vi "Data Display Manager.vi"(6 "Volt Channel":T1={"Index"=[], "Chl Name"=[], "Scale"=[], "Offset"=[], "Sample Rate"=100, "Device Name"="", "Channel"=""}, 7 "Enum":T2=enum."Config Data", 8 "error in":errorcluster, 9 "Raw Data":waveform(dbl)[](array[waveform]), 11 "Data Display Choice":T3) -> (0 "error out":errorcluster, 1 "Overall Mean":dbl[](array[numeric]), 2 "Mean per Second":dbl[](array[numeric]), 3 "VI Ref":refnum<vi>, 4 "Conditioned Data Out":waveform(dbl)[](array[waveform]))   [LabVIEW 2021]
doc: "This Vi has three functions:\nConfig Data - Reset Total Samples, Mean per Second and Overall Mean\nVolt Data - Display Data and calculate Mean per Second and Overall Mean\nDisplay Choice - Choose an appropriate displaying method and pass the chart or graph vi reference out."
uses:
  Control/Data Display Choice Enum.ctl
  Control/Data Display Manager Enum.ctl
  Control/Volt Chl.ctl
  Graph Abstract Class/Pass Ref and Receive Data -- Enum.ctl
  Graph Abstract Class/Graph Data -- cluster.ctl
  Graph Abstract Class/Display Abstract.lvclass
  Chart Class/Chart.lvclass
  Graph Class/Graph.lvclass
  <vilib>/Analysis/baseanly.llb/Mean (DBL).vi
  <vilib>/Analysis/NI_AALBase.lvlib
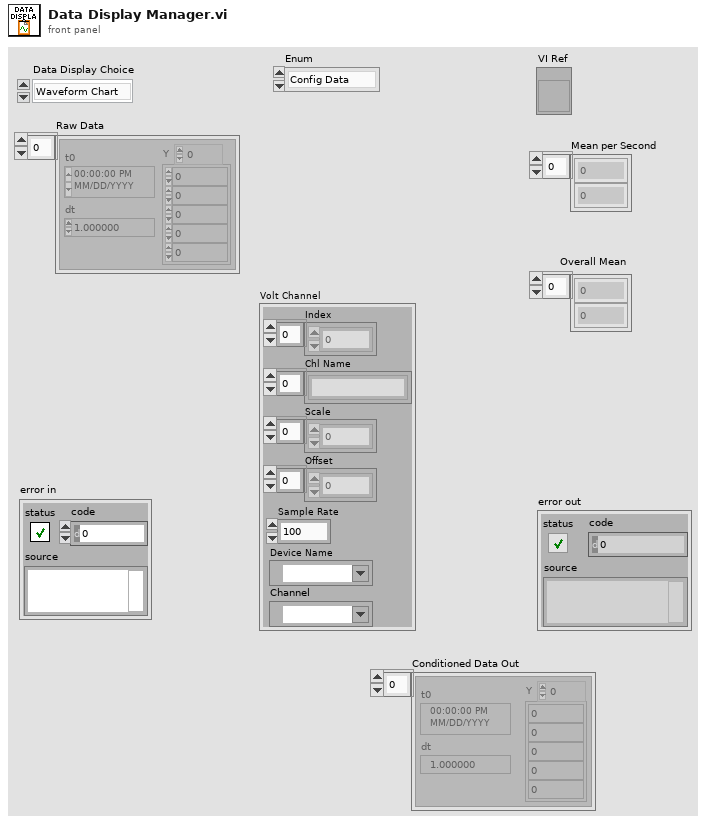
[diagram p1: front panel]
types:
  T1 = typedef "Volt Chl.ctl" = cluster{"Index":i32[], "Chl Name":string[], "Scale":dbl[], "Offset":dbl[], "Sample Rate":i32, "Device Name":tag, "Channel":tag}
  T2 = typedef "Data Display Manager Enum.ctl" = enum16{"Display Choice", "Config Data", "Volt Data"}
  T3 = typedef "Data Display Choice Enum.ctl" = enum16{"Waveform Chart", "Waveform Graph"}
  T4 = typedef "Graph Data -- cluster.ctl" = cluster{"Raw Data":waveform(dbl)[], "Volt Channel":T1}
  T5 = typedef "Pass Ref and Receive Data -- Enum.ctl" = enum16{"Initialize", "Pass Data"}
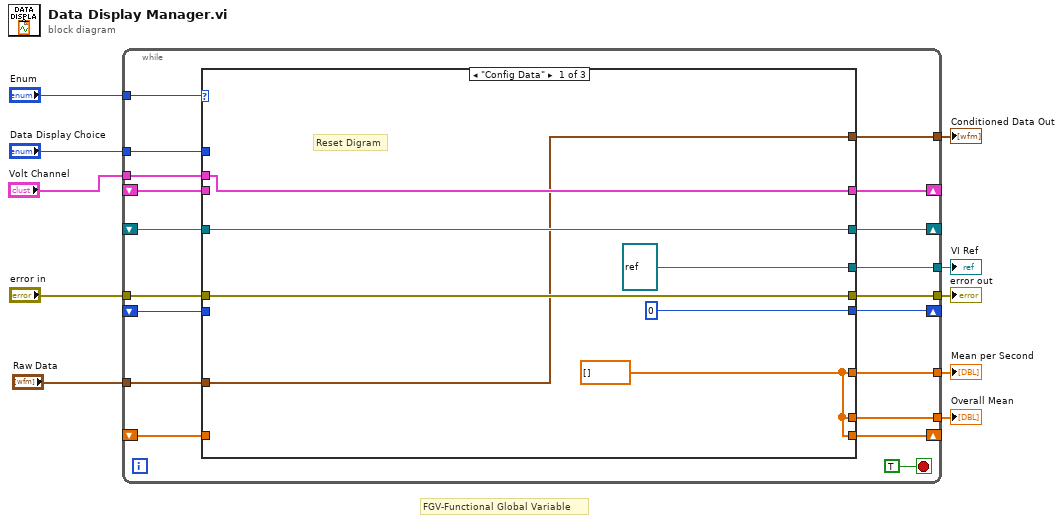
[diagram p0: block diagram]
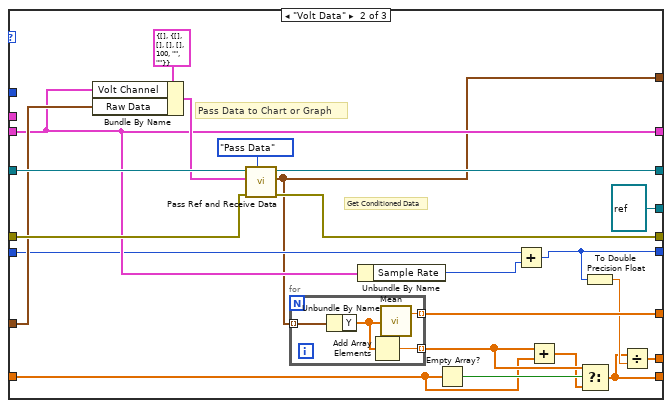
[diagram p2: hidden frame]
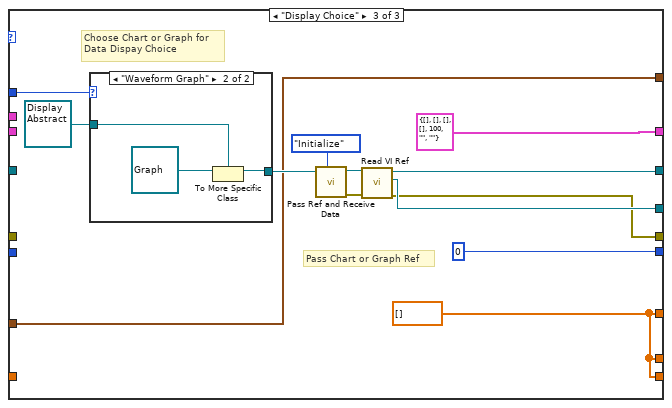
[diagram p3: hidden frame]
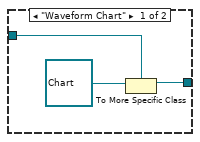
[diagram p4: hidden frame]
diagram:
  # "FGV-Functional Global Variable"
  n1 = while {
    tunnel: "Data Display Choice" -> [w29]
    shift-right: [w27] -> _
    shift-left: _ -> [w23]
    tunnel: [w25] -> w9
    tunnel: "error in" -> [w24]
    tunnel: "Enum" -> [w22]
    shift-right: [w20] -> _
    shift-left: _ -> [w21]
    tunnel: "Raw Data" -> [w19]
    tunnel: "Volt Channel" -> [w18]
    shift-right: [w17] -> _
    shift-left: _ -> [w16]
    tunnel: [w15] -> w2
    shift-right: [w14] -> _
    shift-left: _ -> [w13]
    tunnel: [w12] -> w3
    tunnel: [w26] -> w6
    tunnel: [w11] -> w1
    stop <- TRUE stop-if-true
    n2 = case shown="\"Config Data\"" w22 {
      tunnel: w29 -> [_ _ w74]
      tunnel: [w36 w56 w67] -> w27
      tunnel: [refnum<vi> refnum ("VI Ref") refnum<vi> refnum ("VI Ref") w72] -> w26
      tunnel: [w35 w54 w69] -> w25
      tunnel: w24 -> [w35 w53 _]
      tunnel: w23 -> [w36 w55 _]
      tunnel: w21 -> [_ w49 _]
      tunnel: [w33 w49 T1 {"Index"=[], "Chl Name"=[], "Scale"=[], "Offset"=[], "Sample Rate"=100, "Device Name"="", "Channel"=""} ("Volt Channel")] -> w20
      tunnel: w19 -> [w30 w51 w63]
      tunnel: w18 -> [w33 _ _]
      tunnel: [w32 w39 w65] -> w17
      tunnel: w16 -> [_ w41 _]
      tunnel: [w32 w50 w65] -> w15
      tunnel: [0 w46 0] -> w14
      tunnel: w13 -> [_ w48 _]
      tunnel: [w32 w44 w65] -> w12
      tunnel: [w30 w37 w63] -> w11
      frame "Config Data" {
        w32 = dbl[] []
        # "Reset Digram"
      }
      frame "Volt Data" {
        # "Get Conditioned Data"
        # "Pass Data to Chart or Graph"
        n3 = Bundle By Name(cluster=T4 {"Raw Data"=[], "Volt Channel"={"Index"=[], "Chl Name"=[], "Scale"=[], "Offset"=[], "Sample Rate"=100, "Device Name"="", "Channel"=""}} ("output cluster"), "Volt Channel"=w49, "Raw Data"=w51) -> (w52:T4)
        n4 = call-dynamic "Pass Ref and Receive Data.vi"("Enum State"=Pass_Ref_and_Receive_Data_--_Enum."Pass Data", "error in (no error)"=w53, "Data"=w52, "Graph Manager in"=w55) -> ("error out"=w54:errorcluster, "Data Out"=w37:waveform(dbl)[], "Graph Manager out"=w56:refnum<class "Display Abstract.lvclass">)  [unwired: 5 in]
        n5 = for {
          tunnel: w37 -> [w62] mode=indexing
          tunnel: [w61] -> w50 mode=indexing
          tunnel: [w59] -> w42 mode=indexing
          n6 = Unbundle By Name(w62) -> ("Y"=w60:dbl[])
          n7 = Add Array Elements(numeric array=w60) -> (sum=w59:dbl)
          n8 = call-poly <vilib>:"Mean.vi"("X"=w60) -> ("mean"=w61:dbl)  [unwired: 1 out]
        }
        n9 = Unbundle By Name(w49) -> ("Sample Rate"=w47:i32)
        n10 = Empty Array?(array=w41) -> (empty?=w43:bool)
        n11 = Add(x=w48, y=w47) -> (x+y=w46:i32)
        n12 = Add(x=w42, y=w41) -> (x+y=w40:dbl[])
        n13 = Select(t=w42, s=w43, f=w40) -> (s? t:f=w39:dbl[])
        n14 = To Double Precision Float(number=w46) -> (double precision float=w45:dbl)
        n15 = Divide(x=w39, y=w45) -> (x/y=w44:dbl[])
      }
      frame "Display Choice" {
        w65 = dbl[] []
        # "Pass Chart or Graph Ref"
        # "Choose Chart or Graph for\nData Dispay Choice"
        n16 = case shown="\"Waveform Graph\"" w74 {
          tunnel: refnum<class "Display Abstract.lvclass"> refnum ("Display Abstract.lvclass") -> [w77 w80]
          tunnel: [w76 w79] -> w71
          frame "Waveform Chart" {
            n17 = To More Specific Class(target class=w77, reference=refnum<class "Chart.lvclass"> refnum ("Chart.lvclass")) -> (specific class reference=w76:refnum<class "Display Abstract.lvclass">)  [unwired: 1 in, 1 out]
          }
          frame "Waveform Graph" {
            n18 = To More Specific Class(target class=w80, reference=refnum<class "Graph.lvclass"> refnum ("Graph.lvclass")) -> (specific class reference=w79:refnum<class "Display Abstract.lvclass">)  [unwired: 1 in, 1 out]
          }
        }
        n19 = call-dynamic "Pass Ref and Receive Data.vi"("Enum State"=Pass_Ref_and_Receive_Data_--_Enum."Initialize", "Graph Manager in"=w71) -> ("error out"=w70:errorcluster, "Graph Manager out"=w68:refnum<class "Display Abstract.lvclass">)  [unwired: 7 in, 1 out]
        n20 = call-dynamic "Read VI Ref.vi"("error in (no error)"=w70, "Graph Manager in"=w68) -> ("error out"=w69:errorcluster, "VI Ref"=w72:refnum<vi>, "Graph Manager out"=w67:refnum<class "Display Abstract.lvclass">)  [unwired: 7 in]
      }
    }
  }
  "error out" <- w9
  "VI Ref" <- w6
  "Overall Mean" <- w3
  "Mean per Second" <- w2
  "Conditioned Data Out" <- w1
